vi "Instrument Address.vi"(7 "Command":T1, 8 "error in (no error)":errorcluster, 9 "Data In":string[](array[string]), 10 "path_in":path, 11 "name or relative path":string="AI.ini") -> (0 "error out":errorcluster, 2 "Instrument Parameter":string[][](array[string]), 3 "path_out":path)   [LabVIEW 2021, in "User Interface.lvlib"]
uses:
  User Interface.lvlib
  Instrument Address Command.ctl
  Create Path Command.ctl
  <vilib>/Utility/config.llb/Read Key (String).vi
  <vilib>/Utility/config.llb/Write Key (String).vi
  <vilib>/Utility/config.llb/NI_LVConfig.lvlib
panel:
  in  "Parameter":string[](array[string])
  in  "Instrument Name":string
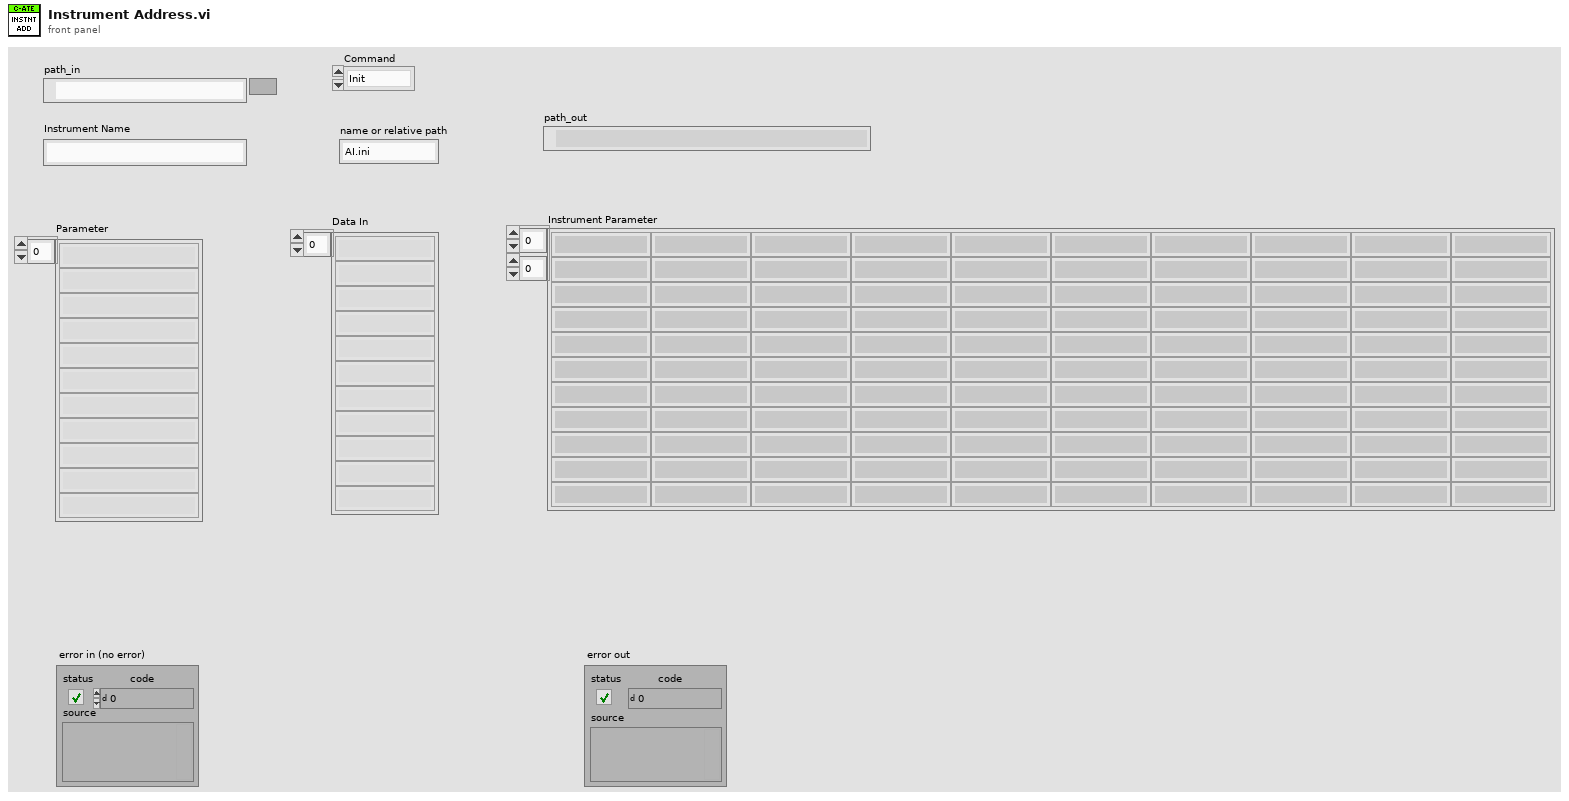
[diagram p1: front panel]
types:
  T1 = typedef "User Interface.lvlib/Instrument Address Command.ctl" = enum16{"Init", "Read", "Write", "Close"}
  T2 = typedef "User Interface.lvlib/Create Path Command.ctl" = enum16{"Authentication", "Hardware", "Configuration", "Calibration", "Instrument", "Test Description", "Serial Data", "Data", "Report", "Action log", "Error Log"}
  T3 = typedef "NI_LVConfig.lvlib/Config Data RefNum.ctl" = refnum<k1>
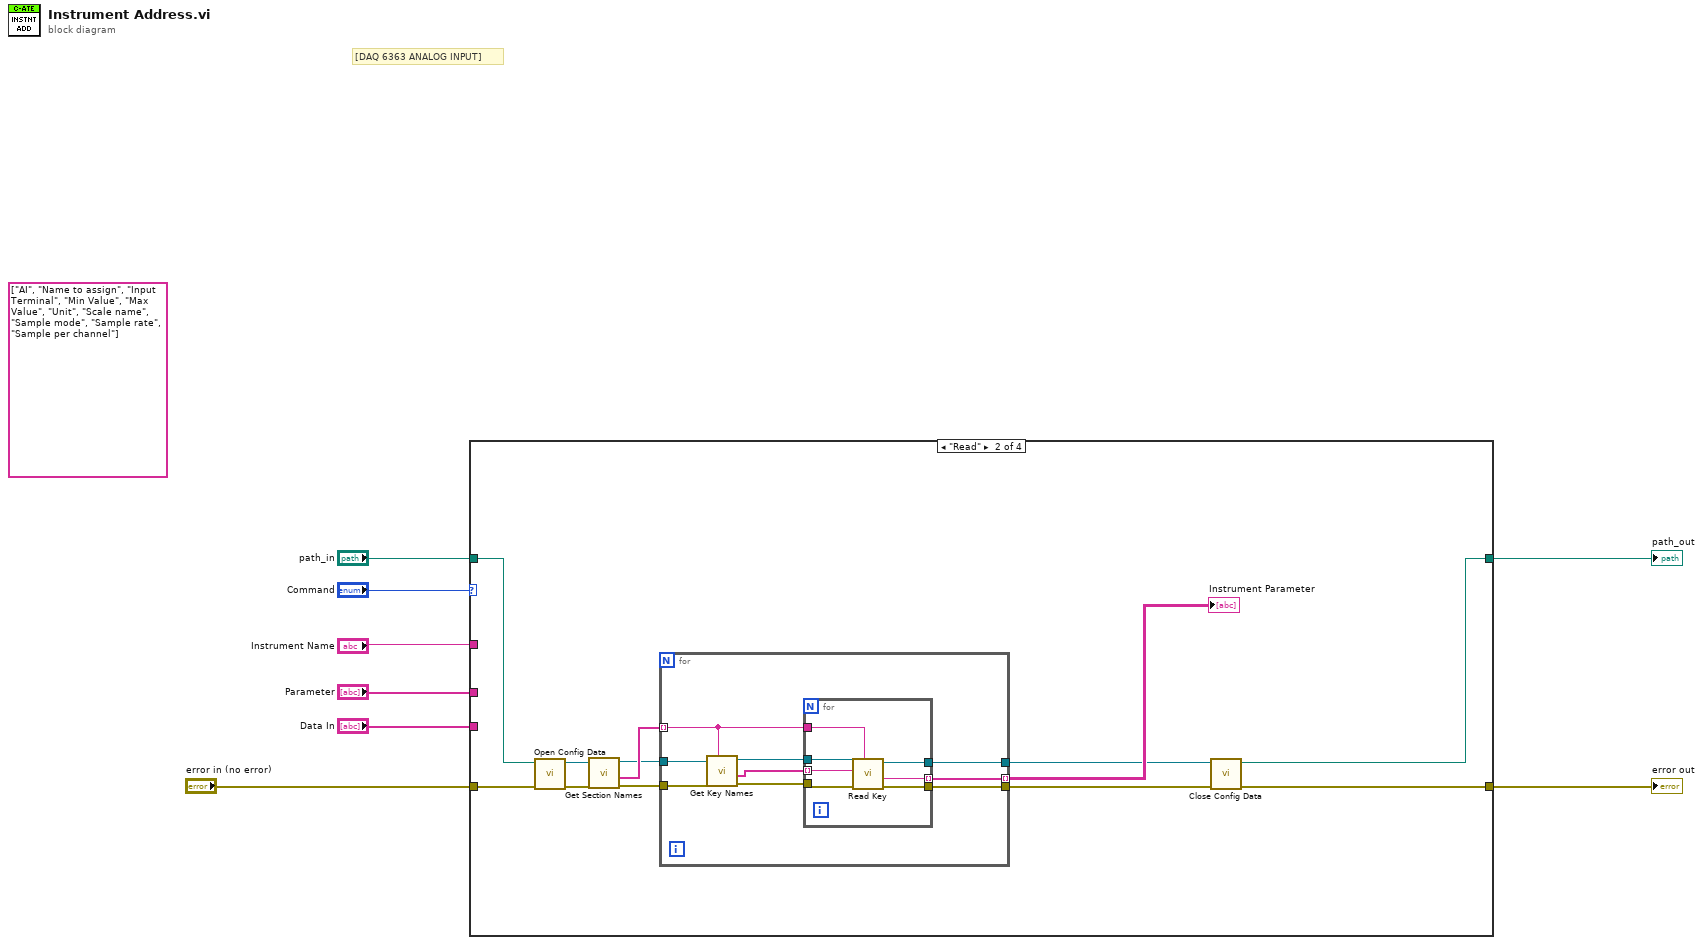
[diagram p0: block diagram]
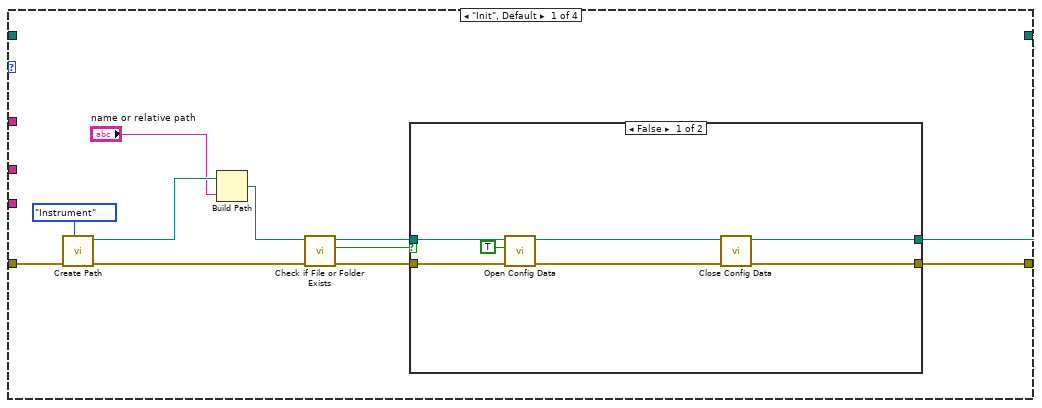
[diagram p2: hidden frame]
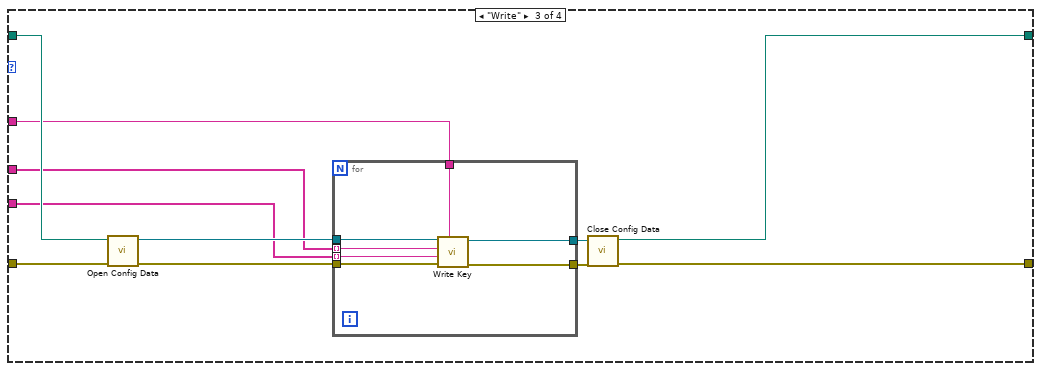
[diagram p4: hidden frame]
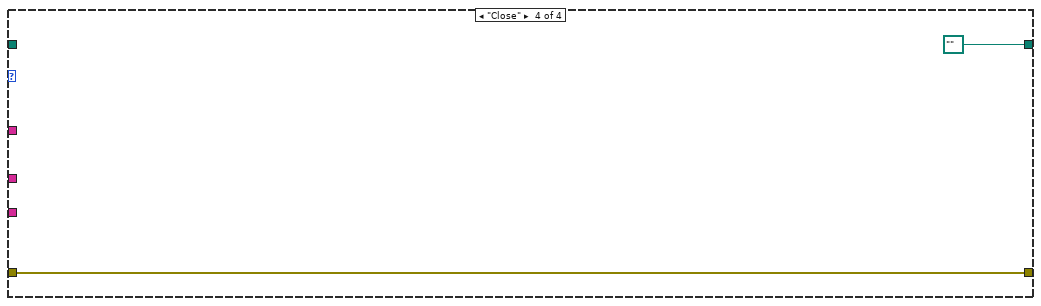
[diagram p5: hidden frame]
diagram:
  (unwired) string[] ["AI", "Name to assign", "Input Terminal", "Min Value", "Max Value", "Unit", "Scale name", "Sample mode", "Sample rate", "Sample per channel"] ("Parameter 2")
  # "[DAQ 6363 ANALOG INPUT]"
  n1 = case shown="\"Read\"" "Command" {
    tunnel: "error in (no error)" -> [w18 w40 w67 w75]
    tunnel: [w10 w39 w62 w75] -> w7
    tunnel: [w9 w37 w60 path "" ("dup path")] -> w5
    tunnel: "path_in" -> [_ w38 w66 _]
    tunnel: "Parameter" -> [_ _ w59 _]
    tunnel: "Data In" -> [_ _ w58 _]
    tunnel: "Instrument Name" -> [_ _ w57 _]
    frame "Init", Default {
      n2 = call "Create Path.vi"("Path Command"=Create_Path_Command."Instrument", "error in (no error)"=w18) -> ("error out"=w14:errorcluster, "created path"=w17:path)  [unwired: 8 in]
      n3 = Build Path(base path=w17, name or relative path="name or relative path") -> (appended path=w15:path)
      n4 = call <vilib>:"Check if File or Folder Exists.vi"("error in (no error)"=w14, "path"=w15) -> ("error out"=w13:errorcluster, "file or folder exists?"=w12:bool, "dup path"=w11:path)  [unwired: 7 in]
      n5 = case shown="False" w12 {
        tunnel: w13 -> [w25 w28]
        tunnel: w11 -> [w26 w27]
        tunnel: [w22 w28] -> w10
        tunnel: [w20 w27] -> w9
        frame False {
          n6 = call <vilib>:"Open Config Data.vi"("error in (no error)"=w25, "create file if necessary (T)"=TRUE, "configuration file path"=w26) -> ("error out"=w23:errorcluster, "refnum"=w21:T3)  [unwired: 6 in, 1 out]
          n7 = call <vilib>:"Close Config Data.vi"("error in (no error)"=w23, "refnum"=w21) -> ("error out"=w22:errorcluster, "file path"=w20:path)  [unwired: 8 in]
        }
        frame True {
        }
      }
    }
    frame "Read" {
      n8 = call <vilib>:"Open Config Data.vi"("error in (no error)"=w40, "configuration file path"=w38) -> ("error out"=w36:errorcluster, "refnum"=w35:T3)  [unwired: 7 in, 1 out]
      n9 = call <vilib>:"Get Section Names.vi"("error in (no error)"=w36, "refnum"=w35) -> ("error out"=w34:errorcluster, "section names"=w33:string[], "refnum out"=w29:T3)  [unwired: 7 in]
      n10 = for {
        tunnel: w34 -> [w49]
        tunnel: w33 -> [w46] mode=indexing
        tunnel: [w45] -> w32 mode=indexing
        tunnel: [w44] -> w31
        tunnel: [w42] -> w30
        tunnel: w29 -> [w41]
        n11 = call <vilib>:"Get Key Names.vi"("section"=w46, "error in (no error)"=w49, "refnum"=w41) -> ("error out"=w48:errorcluster, "key names"=w47:string[], "refnum out"=w43:T3)  [unwired: 5 in, 1 out]
        n12 = for {
          tunnel: w48 -> [w54]
          tunnel: w47 -> [w56] mode=indexing
          tunnel: w46 -> [w55]
          tunnel: [w53] -> w44
          tunnel: [w52] -> w45 mode=indexing
          tunnel: w43 -> [w51]
          tunnel: [w50] -> w42
          n13 = call-poly <vilib>:"Read Key.vi"("section"=w55, "error in (no error)"=w54, "key"=w56, "refnum"=w51) -> ("error out"=w53:errorcluster, "value"=w52:string, "refnum out"=w50:T3)  [unwired: 4 in, 1 out]
        }
      }
      "Instrument Parameter" <- w32
      n14 = call <vilib>:"Close Config Data.vi"("error in (no error)"=w31, "refnum"=w30) -> ("error out"=w39:errorcluster, "file path"=w37:path)  [unwired: 8 in]
    }
    frame "Write" {
      n15 = call <vilib>:"Open Config Data.vi"("error in (no error)"=w67, "configuration file path"=w66) -> ("error out"=w65:errorcluster, "refnum"=w64:T3)  [unwired: 7 in, 1 out]
      n16 = for {
        tunnel: w65 -> [w74]
        tunnel: w64 -> [w73]
        tunnel: [w72] -> w63
        tunnel: [w71] -> w61
        tunnel: w59 -> [w70] mode=indexing
        tunnel: w58 -> [w69] mode=indexing
        tunnel: w57 -> [w68]
        n17 = call-poly <vilib>:"Write Key.vi"("section"=w68, "error in (no error)"=w74, "value"=w69, "key"=w70, "refnum"=w73) -> ("error out"=w72:errorcluster, "refnum out"=w71:T3)  [unwired: 4 in, 1 out]
      }
      n18 = call <vilib>:"Close Config Data.vi"("error in (no error)"=w63, "refnum"=w61) -> ("error out"=w62:errorcluster, "file path"=w60:path)  [unwired: 8 in]
    }
    frame "Close" {
    }
  }
  "error out" <- w7
  "path_out" <- w5
